vi "read project file.vi"(8 "error in (no error)":errorcluster, 10 "lookup in":variant, 11 "Path":path) -> (0 "error out":errorcluster, 2 "lookup out":variant)   [LabVIEW 2014]
uses:
  <vilib>/xml/Load XML File.vi
  <vilib>/xml/Close Reference(Node).vi
  <vilib>/xml/NI_XML.lvlib
  <resource>/objmgr/DOMUserDefRef.rc
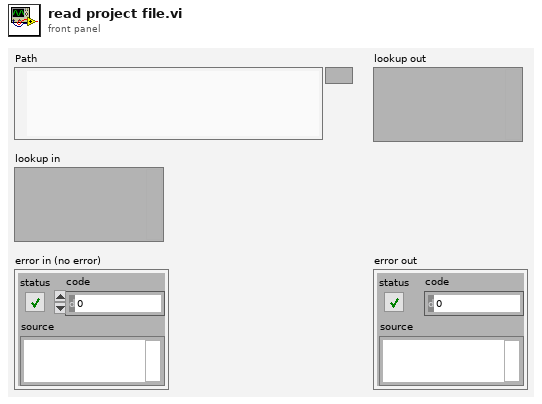
[diagram p1: front panel]
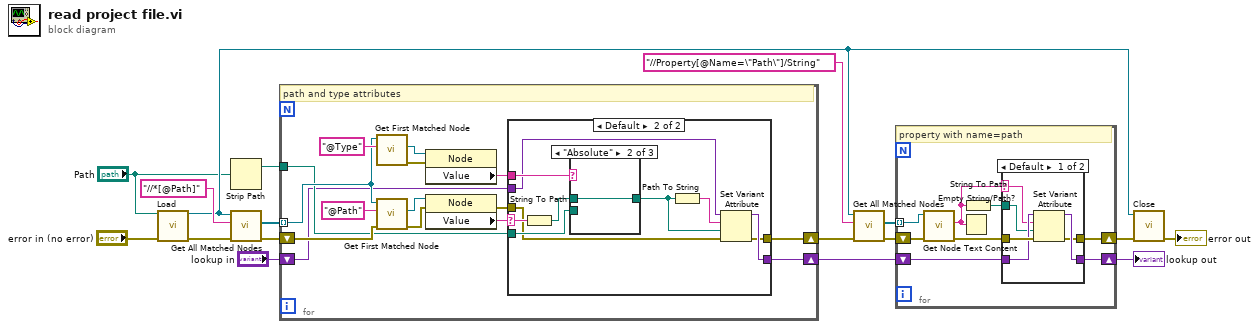
[diagram p0: block diagram]
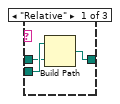
[diagram p4: hidden frame]
diagram:
  n1 = call-poly <vilib>:"Load.vi"("path to XML document"="Path", "error in (no error)"="error in (no error)") -> ("DOM document out"=w9:refnum<k20>, "error out"=w15:errorcluster)  [unwired: 11 in, 1 out]
  n2 = Strip Path(path="Path") -> (stripped path=w4:path)  [unwired: 1 out]
  n3 = call <vilib>:"Get All Matched Nodes.vi"("error in (no error)"=w15, "XPath expression"="//*[@Path]", "node in"=w9) -> ("error out"=w12:errorcluster, "node result array"=w13:refnum<k20>[])  [unwired: 6 in, 1 out]
  n4 = for {
    tunnel: w13 -> [w24] mode=indexing
    shift-right: [w19] -> w7
    shift-left: w12 -> [w32]
    tunnel: w4 -> [w22]
    shift-right: [w21] -> w2
    shift-left: "lookup in" -> [w20]
    # "path and type attributes"
    n5 = call <vilib>:"Get First Matched Node.vi"("XPath expression"="@Type", "node in"=w24) -> ("error out"=w26:errorcluster, "node result"=w27:refnum<k20>)  [unwired: 7 in, 1 out]
    n6 = call <vilib>:"Get First Matched Node.vi"("error in (no error)"=w32, "XPath expression"="@Path", "node in"=w24) -> ("error out"=w30:errorcluster, "node result"=w29:refnum<k20>)  [unwired: 6 in, 1 out]
    n7 = property class="Node"(reference=w27, error in=w26) -> ("Value"=w23:string)  [unwired: 2 out]
    n8 = property class="Node"(reference=w29, error in=w30) -> (error out=w18:errorcluster, "Value"=w28:string)  [unwired: 1 out]
    n9 = case shown="Default" w28 {
      selector: w28 -> [_ w44]
      tunnel: w23 -> [_ w43]
      tunnel: w22 -> [_ w41]
      tunnel: [w34 w37] -> w21
      tunnel: w20 -> [w34 w40]
      tunnel: [w33 w36] -> w19
      tunnel: w18 -> [w33 w35]
      frame "\u0000" {
      }
      frame Default {
        n10 = String To Path(string=w44) -> (path=w42:path)
        n11 = case shown="\"Absolute\"" w43 {
          tunnel: [w46 w48 w49] -> w38
          tunnel: w42 -> [w45 w48 w49]
          tunnel: w41 -> [w47 _ _]
          frame "Relative" {
            n12 = Build Path(base path=w47, name or relative path=w45) -> (appended path=w46:path)
          }
          frame "Absolute" {
          }
          frame "\u0000", Default {
          }
        }
        n13 = Path To String(path=w38) -> (string=w39:string)
        n14 = Set Variant Attribute(Variant=w40, name=w39, value=w38, error in=w35) -> (Variant out=w37:variant, error out=w36:errorcluster)  [unwired: 1 out]
      }
    }
  }
  n15 = call <vilib>:"Get All Matched Nodes.vi"("error in (no error)"=w7, "XPath expression"="//Property[@Name=\"Path\"]/String", "node in"=w9) -> ("error out"=w11:errorcluster, "node result array"=w10:refnum<k20>[])  [unwired: 6 in, 1 out]
  n16 = for {
    tunnel: w10 -> [w56] mode=indexing
    shift-right: [w54] -> w6
    shift-left: w11 -> [w57]
    shift-right: [w51] -> w1
    shift-left: w2 -> [w52]
    # "property with name=path"
    n17 = call <vilib>:"Get Node Text Content.vi"("error in (no error)"=w57, "node in"=w56) -> ("error out"=w53:errorcluster, "node text"=w55:string)  [unwired: 7 in, 1 out]
    n18 = Empty String/Path?(string/path=w55) -> ()  [unwired: 1 out]
    n19 = String To Path(string=w55) -> (path=w50:path)
    n20 = case shown="Default" w55 {
      selector: w55 -> [w59 _]
      tunnel: [w62 w65] -> w54
      tunnel: w53 -> [w61 w65]
      tunnel: w52 -> [w60 w64]
      tunnel: [w63 w64] -> w51
      tunnel: w50 -> [w58 _]
      frame Default {
        n21 = Set Variant Attribute(Variant=w60, name=w59, value=w58, error in=w61) -> (Variant out=w63:variant, error out=w62:errorcluster)  [unwired: 1 out]
      }
      frame "\u0000" {
      }
    }
  }
  "lookup out" <- w1
  n22 = call-poly <vilib>:"Close.vi"("error in (no error)"=w6, "node"=w9) -> ("error out"=→"error out":errorcluster)  [unwired: 7 in]
